vi "Acquire data.vi"(8 "error in":errorcluster, 11 "Run info":T4) -> (0 "error out":errorcluster, 2 "Data out":T1, 3 "Run info out":T4)   [LabVIEW 2012]
uses:
  Run info.ctl
  Data.ctl
  Treatment.ctl
  Treatment type.ctl
  <vilib>/DAQmx/read.llb/DAQmx Read (Analog 2D DBL NChan NSamp).vi
  <vilib>/DAQmx/miscellaneous.llb/DAQmx Fill In Error Info.vi
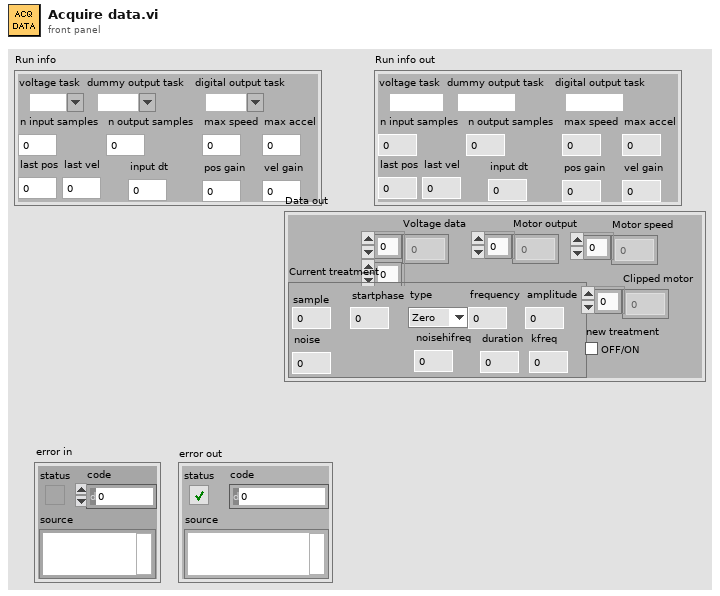
[diagram p1: front panel]
types:
  T1 = typedef "Data.ctl" = cluster{"Voltage data":dbl[][], "Motor output":dbl[], "Current treatment":T2, "Motor speed":dbl[], "Clipped motor":dbl[], "new treatment":bool}
  T2 = typedef "Treatment.ctl" = cluster{"sample":dbl, "startphase":dbl, "type":T3, "frequency":dbl, "amplitude":dbl, "noise":dbl, "duration":dbl, "kfreq":dbl, "noisehifreq":dbl}
  T3 = typedef "Treatment type.ctl" = enum16{"Zero", "Sine", "Frequency sweep"}
  T4 = typedef "Run info.ctl" = cluster{"voltage task":refnum<k21>, "dummy output task":refnum<k21>, "digital output task":refnum<k21>, "n input samples":i32, "n output samples":i32, "max speed":dbl, "max accel":dbl, "last pos":dbl, "last vel":dbl, "pos gain":dbl, "vel gain":dbl, "input dt":dbl}
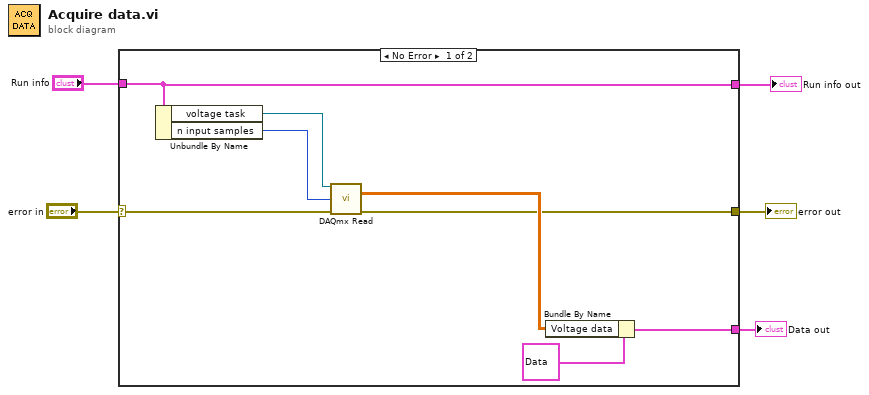
[diagram p0: block diagram]
diagram:
  n1 = case shown="No Error" "error in" {
    selector: "error in" -> [w13 w14]
    tunnel: "Run info" -> [w7 w15]
    tunnel: [w8 w14] -> w3
    tunnel: [w7 w15] -> w2
    tunnel: [w6 _] -> w1
    frame No Error {
      n2 = Unbundle By Name(w7) -> ("voltage task"=w12:refnum<k21>, "n input samples"=w11:i32)
      n3 = call-poly <vilib>:"DAQmx Read.vi"("task/channels in"=w12, "number of samples per channel"=w11, "error in"=w13) -> ("data"=w9:dbl[][], "error out"=w8:errorcluster)  [unwired: 10 in, 1 out]
      n4 = Bundle By Name(cluster=T1 {"Voltage data"=[], "Motor output"=[], "Current treatment"={"sample"=0.0, "startphase"=0.0, "type"=enum."Zero", "frequency"=0.0, "amplitude"=0.0, "noise"=0.0, "duration"=0.0, "kfreq"=0.0, "noisehifreq"=0.0}, "Motor speed"=[], "Clipped motor"=[], "new treatment"=FALSE} ("Data out"), "Voltage data"=w9) -> (w6:T1)
    }
    frame Error {
    }
  }
  "Data out" <- w1
  "Run info out" <- w2
  "error out" <- w3
